vi "App_Training Mode Initialize.vi"(8 "error in":errorcluster, 11 "VI Reference":refnum<vi>) -> (0 "error out":errorcluster, 3 "Event Registration Refnum":refnum<event-registration>)   [LabVIEW 2015, in "Application 1.lvlib"]
uses:
  Application 1.lvlib
  Data Def/App_User Event Data.ctl
  Data Def/App_User Event Method.ctl
  Data Def/App_Subpanel Name.ctl
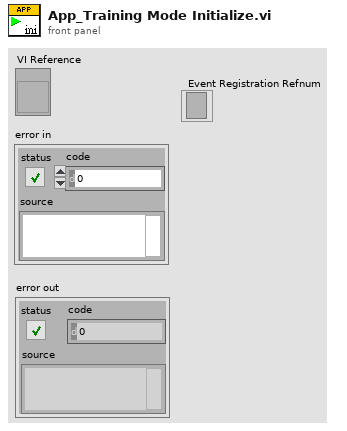
[diagram p1: front panel]
types:
  T1 = typedef "Application 1.lvlib/App_Subpanel Name.ctl" = enum16{"Main", "Menu", "User Registering", "User Setting", "Monitor", "Traning Mode", "Query Data", "Connect Setting"}
  T2 = typedef "Application 1.lvlib/App_User Event Data.ctl" = cluster{"Command":string, "Data":variant}
  T3 = typedef "Application 1.lvlib/App_User Event Method.ctl" = enum16{"Initialize", "Put Event", "Get Ref.", "Release"}
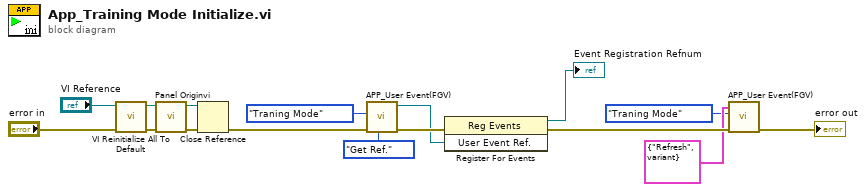
[diagram p0: block diagram]
diagram:
  n1 = call "VI Reinitialize All To Default.vi"("error in"="error in", "VI Reference in"="VI Reference") -> ("error out"=w16:errorcluster, "VI Reference out"=w15:refnum<vi>)  [unwired: 8 in]
  n2 = call "Panel Originvi.vi"("error in"=w16, "VI Reference In"=w15) -> ("error out"=w13:errorcluster, "VI Reference Out"=w12:refnum<vi>)  [unwired: 8 in]
  n3 = Close Reference(reference=w12, error in (no error)=w13) -> (error out=w11:errorcluster)
  n4 = call "APP_User Event(FGV).vi"("User Event Method(Put Event)"=App_User_Event_Method."Get Ref." ("User Event Method"), "error in"=w11, "Subpanel Name"=App_Subpanel_Name."Traning Mode") -> ("error out"=w8:errorcluster, "User Event Ref."=w7:refnum<user-event>)  [unwired: 7 in]
  n5 = register-events(error in=w8, w7) -> (reference out=→"Event Registration Refnum":refnum<event-registration>, error out=w4:errorcluster)  [unwired: 1 in]
  n6 = call "APP_User Event(FGV).vi"("error in"=w4, "Subpanel Name"=App_Subpanel_Name."Traning Mode", "User Event Data"=T2 {"Command"="Refresh", "Data"=variant}) -> ("error out"=→"error out":errorcluster)  [unwired: 7 in, 1 out]
